vi "Set Channels.vi"(8 "error in":errorcluster, 10 "Channels":T1[](array[typedef]) format="%.0x", 11 "Execution Unit":T2 {"ReadWrite Channels" format="%.0x"; "Outgoing Channels" format="%.0x"; "Incoming Channels" format="%.0x"}) -> (0 "error out":errorcluster, 3 "Execution Unit out":T2 {"ReadWrite Channels" format="%.0x"; "Outgoing Channels" format="%.0x"; "Incoming Channels" format="%.0x"})   [LabVIEW 2020, in "Ballard ARINC 429 Engine.lvlib" / "Interfaces.lvlib"]
uses:
  Interfaces.lvlib
  Controls/Execution Unit Information.ctl
  Execution Unit/Execution Unit.lvclass
  <vilib>/NI VeriStand/Custom Device API/Custom Device Item Ref.ctl
  <vilib>/NI VeriStand/Custom Device API/Custom Device API.lvlib
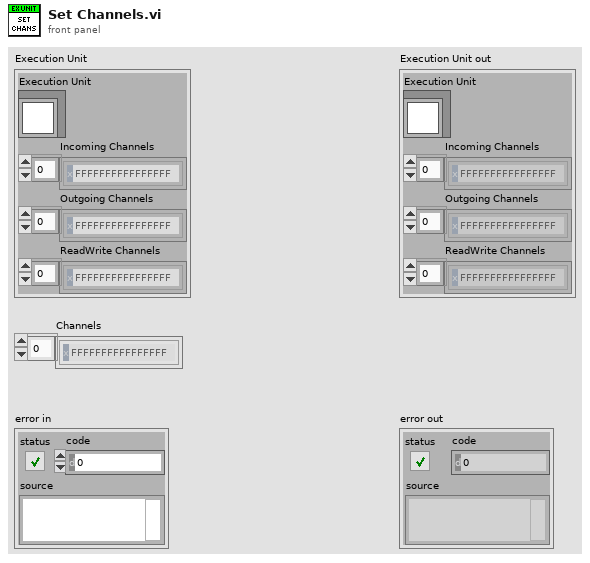
[diagram p1: front panel]
types:
  T1 = typedef "Custom Device API.lvlib/Custom Device Item Ref.ctl" = u64
  T2 = typedef "Ballard ARINC 429 Engine.lvlib/Interfaces.lvlib/Execution Unit Information.ctl" = cluster{"Execution Unit":refnum<class "Execution Unit.lvclass">, "Incoming Channels":T1[], "Outgoing Channels":T1[], "ReadWrite Channels":T1[]}
  T3 = typedef "Custom Device API.lvlib/Custom Device Channel.ctl" = cluster{"Type":T4, "Units":string, "Default Value":dbl, "Faultable":bool, "Scalable":bool}
  T4 = typedef "Custom Device API.lvlib/Custom Device Channel Type.ctl" = enum16{"Input", "Output"}
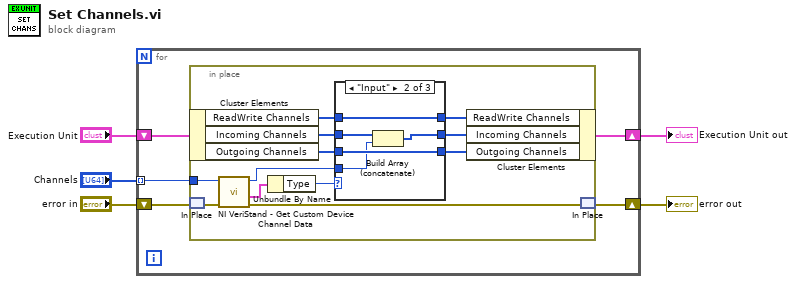
[diagram p0: block diagram]
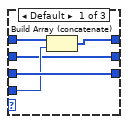
[diagram p2: hidden frame]
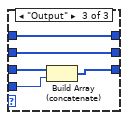
[diagram p3: hidden frame]
diagram:
  n1 = for {
    tunnel: "Channels" -> [w9] mode=indexing
    shift-right: [w6] -> w1
    shift-left: "Execution Unit" -> [w10]
    shift-right: [w7] -> w2
    shift-left: "error in" -> [w8]
    n2 = in-place {
      in-place-border: w9 -> [w22]
      n3 = in-place-cluster #1(w10) -> ("ReadWrite Channels"=w12:T1[], "Incoming Channels"=w20:T1[], "Outgoing Channels"=w19:T1[])
      n4 = in-place-match #2(w8) -> (w18:errorcluster)
      n5 = call <vilib>:"NI VeriStand - Get Custom Device Channel Data.vi"("error in (no error)"=w18, "Channel Ref in"=w22) -> ("error out"=w13:errorcluster, "Channel"=w21:T3, "Channel Ref out"=w16:T1)  [unwired: 4 in, 3 out]
      n6 = Unbundle By Name(w21) -> ("Type"=w17:T4)
      n7 = case shown="\"Input\"" w17 {
        tunnel: w20 -> [w23 w32 w36]
        tunnel: w19 -> [w27 w31 w37]
        tunnel: w16 -> [w26 w30 w35]
        tunnel: [w23 w29 w36] -> w15
        tunnel: [w27 w31 w34] -> w14
        tunnel: w12 -> [w24 w28 w33]
        tunnel: [w25 w28 w33] -> w11
        frame Default {
          n8 = Build Array (concatenate)(w24, w26) -> (w25:T1[])
        }
        frame "Input" {
          n9 = Build Array (concatenate)(w32, w30) -> (w29:T1[])
        }
        frame "Output" {
          n10 = Build Array (concatenate)(w37, w35) -> (w34:T1[])
        }
      }
      n11 = in-place-cluster #1("ReadWrite Channels"=w11, "Incoming Channels"=w15, "Outgoing Channels"=w14) -> (w6:T2)
      n12 = in-place-match #2(w13) -> (w7:errorcluster)
    }
  }
  "Execution Unit out" <- w1
  "error out" <- w2
